vi "WPI_CANJaguar_GetStatus.vi"(8 "error in (no error)":errorcluster, 9 "Force On-Demand":bool, 10 "Status Select":T1[](array[typedef])=[enum."Output Voltage"], 11 "CAN Jaguar Ref":T3={"DeviceStatus"={"status"=FALSE, "code"=0, "source"=""}, "Type"=enum."PWM", "PWM"={"PWM Channel"=enum."PWM 1", "DeadBand"={"Name"="", "maxPositivePwm"=0, "minPositivePwm"=0, "centerPwm"=0, "maxNegativePwm"=0, "minNegativePwm"=0, "angularRange"=0}}, "CAN"={"Device Number"=0, "SetOutput VI Ref"=variant(enum8{"Percent VBus", "Current", "Speed", "Position", "Voltage"} enum."Percent VBus"), "GetOutput VI Ref"=variant(refnum<k1> refnum), "Enable VI Ref"=variant(dbl 12.0), "Disable VI Ref"=variant(enum8{"Percent VBus", "Speed", "Position", "Slave", "Unchanged / Invalid", "Voltage Compensation", "Current", "Motion Profile"} enum."Percent VBus"), "Data"=variant}, "Invert"=FALSE}) -> (0 "error out":errorcluster, 2 "Status":T2 {"Fault Counters"."CAN Status" format="%.0x"}, 3 "CAN Jaguar Ref":T3={"DeviceStatus"={"status"=FALSE, "code"=0, "source"=""}, "Type"=enum."PWM", "PWM"={"PWM Channel"=enum."PWM 1", "DeadBand"={"Name"="", "maxPositivePwm"=0, "minPositivePwm"=0, "centerPwm"=0, "maxNegativePwm"=0, "minNegativePwm"=0, "angularRange"=0}}, "CAN"={"Device Number"=0, "SetOutput VI Ref"=variant(enum8{"Percent VBus", "Current", "Speed", "Position", "Voltage"} enum."Percent VBus"), "GetOutput VI Ref"=variant(refnum<k1> refnum), "Enable VI Ref"=variant(dbl 12.0), "Disable VI Ref"=variant(enum8{"Percent VBus", "Speed", "Position", "Slave", "Unchanged / Invalid", "Voltage Compensation", "Current", "Motion Profile"} enum."Percent VBus"), "Data"=variant}, "Invert"=FALSE})   [LabVIEW 2016]
doc: "Read status information from a CAN Jaguar.\n\nThis VI allows you to specify which parts of the status you care about so that you do not waste CAN bus bandwidth. Use this VI to read status <B>On Demand</B> or status that is already received on a <B>Periodic Status Channel</B>.\n\nAll outputs are in engineering units (Volts, Amps, degrees Celsius, Rotations, and Rotations per Minute)\n\nSticky outputs are faults or limits that have occurred since the last time they were read, but may not be the current condition."
uses:
  <vilib>/Rock Robotics/WPI/MotorControl/WPI_MotorControlDeviceRef.ctl
  <vilib>/Rock Robotics/WPI/MotorControl/WPI_MotorControlType.ctl
  <vilib>/Rock Robotics/SystemInterfaces/DIO/FPGA_DIOPWMChannel.ctl
  <vilib>/Rock Robotics/WPI/PWM/WPI_PWMDeadband.ctl
  <vilib>/Rock Robotics/WPI/ThirdParty/CanMotor/CAN Jaguar/SubVIs/WPI_CANJaguar_Status.ctl
  <vilib>/Rock Robotics/WPI/ThirdParty/CanMotor/CAN Jaguar/SubVIs/WPI_CANJaguar_StatusSelect.ctl
  <vilib>/Rock Robotics/WPI/ThirdParty/CanMotor/CAN Jaguar/SubVIs/WPI_CANJaguar_StatusChannelSelect.ctl
  <vilib>/Rock Robotics/WPI/ThirdParty/CanMotor/CAN Jaguar/SubVIs/WPI_CAN_SystemMessageIDs.ctl
  <vilib>/Rock Robotics/WPI/ThirdParty/CanMotor/CAN Jaguar/SubVIs/WPI_CAN_MotorMessageIDs.ctl
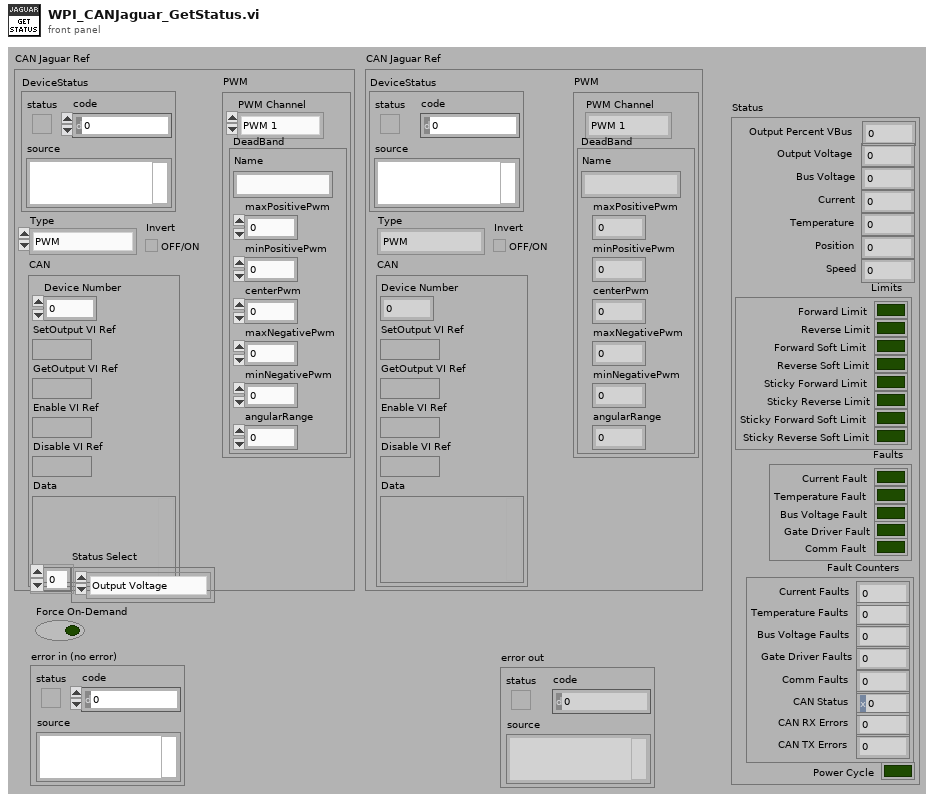
[diagram p1: front panel]
types:
  T1 = typedef "WPI_CANJaguar_StatusSelect.ctl" = enum16{"Output Percent VBus", "Output Voltage", "Bus Voltage", "Current", "Temperature", "Position", "Speed", "Limit Switches", "Faults", "Fault Counters", "Power Cycle"}
  T2 = typedef "WPI_CANJaguar_Status.ctl" = cluster{"Output Percent VBus":dbl, "Output Voltage":dbl, "Bus Voltage":dbl, "Current":dbl, "Temperature":dbl, "Position":dbl, "Speed":dbl, "Limits":cluster{"Forward Limit":bool, "Reverse Limit":bool, "Forward Soft Limit":bool, "Reverse Soft Limit":bool, "Sticky Forward Limit":bool, "Sticky Reverse Limit":bool, "Sticky Forward Soft Limit":bool, "Sticky Reverse Soft Limit":bool}, "Faults":cluster{"Current Fault":bool, "Temperature Fault":bool, "Bus Voltage Fault":bool, "Gate Driver Fault":bool, "Comm Fault":bool}, "Fault Counters":cluster{"Current Faults":u8, "Temperature Faults":u8, "Bus Voltage Faults":u8, "Gate Driver Faults":u8, "Comm Faults":u8, "CAN Status":u8, "CAN RX Errors":u8, "CAN TX Errors":u8}, "Power Cycle":bool}
  T3 = typedef "WPI_MotorControlDeviceRef.ctl" = cluster{"DeviceStatus":errorcluster, "Type":T4, "PWM":cluster{"PWM Channel":T5, "DeadBand":T6}, "CAN":cluster{"Device Number":u8, "SetOutput VI Ref":variant, "GetOutput VI Ref":variant, "Enable VI Ref":variant, "Disable VI Ref":variant, "Data":variant}, "Invert":bool}
  T4 = typedef "WPI_MotorControlType.ctl" = enum16{"PWM", "CAN"}
  T5 = typedef "FPGA_DIOPWMChannel.ctl" = enum8{"PWM 0", "PWM 1", "PWM 2", "PWM 3", "PWM 4", "PWM 5", "PWM 6", "PWM 7", "PWM 8", "PWM 9", "PWM MXP 0", "PWM MXP 1", "PWM MXP 2", "PWM MXP 3", "PWM MXP 4", "PWM MXP 5", "PWM MXP 6", "PWM MXP 7", "PWM MXP 8", "PWM MXP 9", "Invalid"}
  T6 = typedef "WPI_PWMDeadband.ctl" = cluster{"Name":string, "maxPositivePwm":i32, "minPositivePwm":i32, "centerPwm":i32, "maxNegativePwm":i32, "minNegativePwm":i32, "angularRange":u16}
  T7 = typedef "WPI_CANJaguar_StatusChannelSelect.ctl" = enum16{"Periodic Status Channel 1", "Periodic Status Channel 2", "Periodic Status Channel 3", "Periodic Status Channel 4", "On Demand Status"}
  T8 = enum16{"big-endian, network order", "native, host order", "little-endian"}
  T9 = typedef "WPI_CAN_PeriodicStatusIDs.ctl" = enum16{"Disabled", "Percent VBus Out (Byte 0)", "Percent VBus Out (Byte 1)", "VBus (Byte 0)", "VBus (Byte 1)", "Current (Byte 0)", "Current (Byte 1)", "Temperature (Byte 0)", "Temperature (Byte 1)", "Position (Byte 0)", "Position (Byte 1)", "Position (Byte 2)", "Position (Byte 3)", "Speed (Byte 0)", "Speed (Byte 1)", "Speed (Byte 2)", "Speed (Byte 3)", "Limit Switches (No Clear)", "Limit Switches (Clear)", "Faults", "Sticky Faults (No Clear)", "Sticky Faults (Clear)", "Volts Out (Byte 0)", "Volts Out (Byte 1)", "Current Fault Counter", "Temperature Fault Counter", "VBus Fault Counter", "Gate Driver Fault Counter", "Comm Fault Counter", "CANSTS", "CANERR (Byte 0)", "CANERR (Byte 1)", "Power Cycle"}
  T10 = typedef "WPI_CAN_SystemMessageIDs.ctl" = u32
  T11 = typedef "WPI_CAN_MotorMessageIDs.ctl" = u32
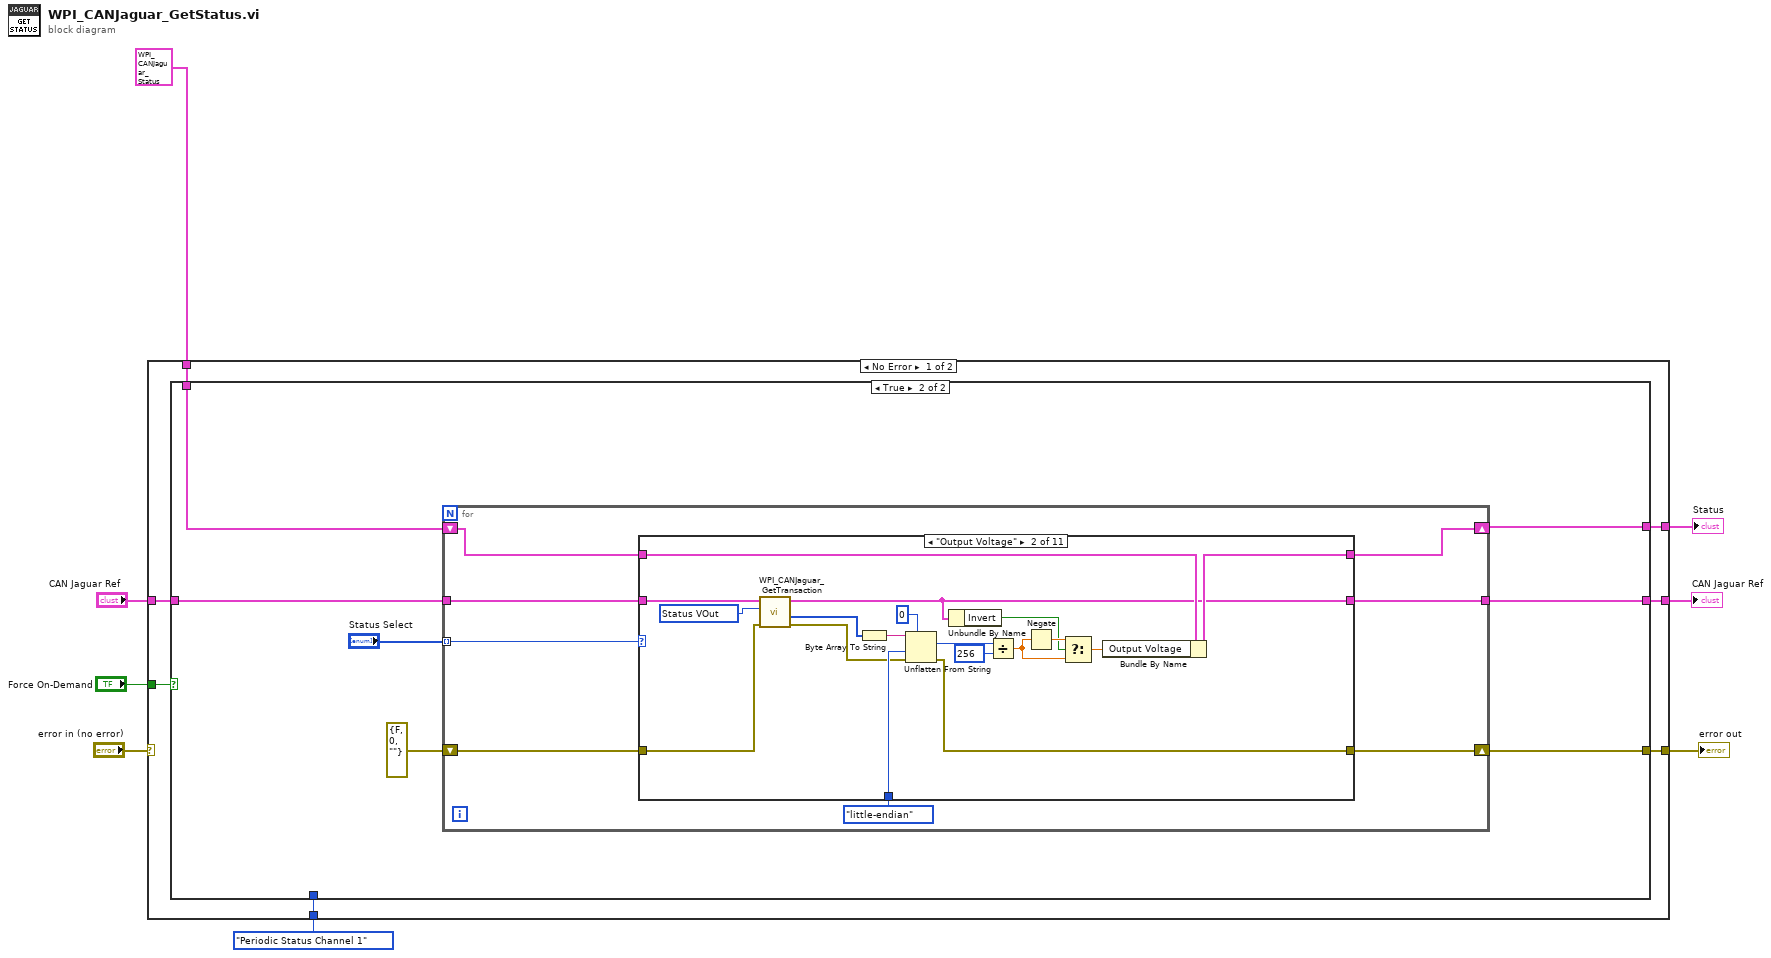
[diagram p0: block diagram]
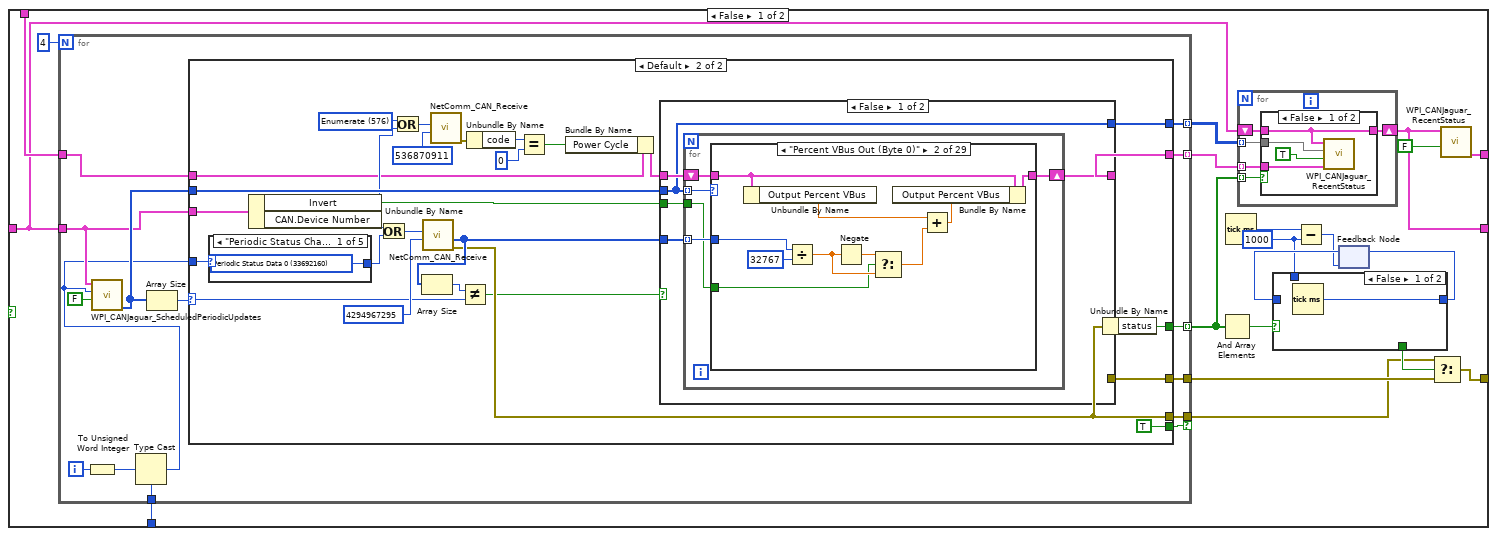
[diagram p2: hidden frame]
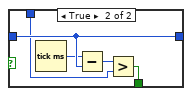
[diagram p3: hidden frame]
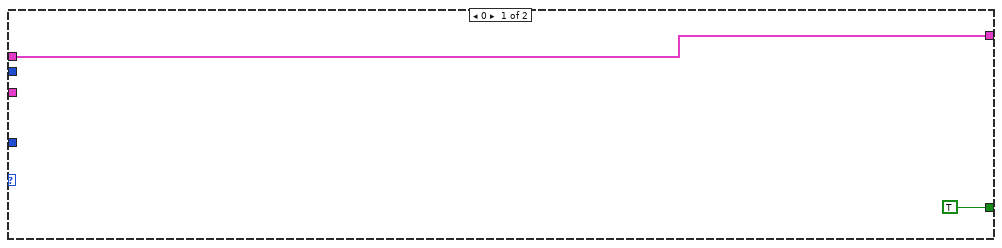
[diagram p5: hidden frame]
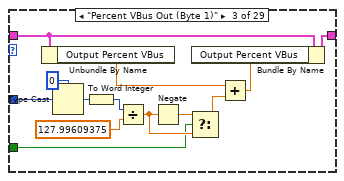
[diagram p7: hidden frame]
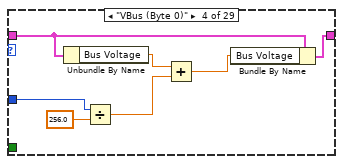
[diagram p8: hidden frame]
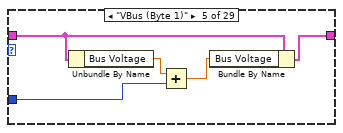
[diagram p9: hidden frame]
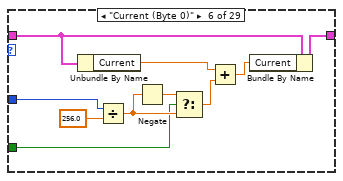
[diagram p10: hidden frame]
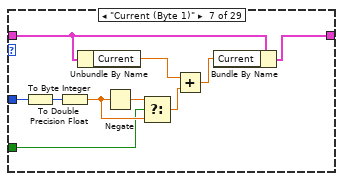
[diagram p11: hidden frame]
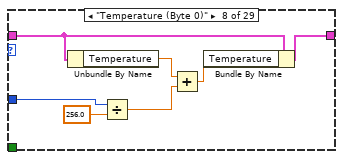
[diagram p12: hidden frame]
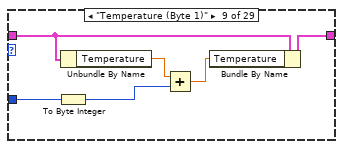
[diagram p13: hidden frame]
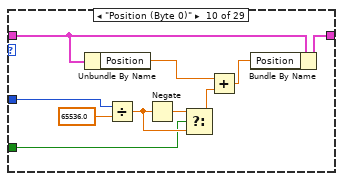
[diagram p14: hidden frame]
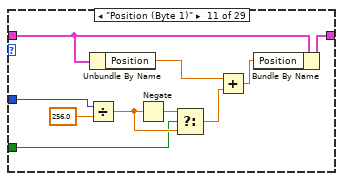
[diagram p15: hidden frame]
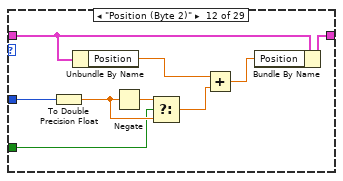
[diagram p16: hidden frame]
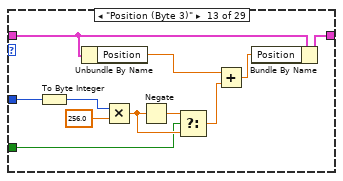
[diagram p17: hidden frame]
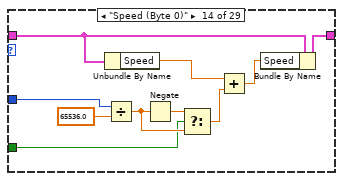
[diagram p18: hidden frame]
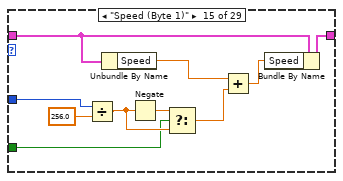
[diagram p19: hidden frame]
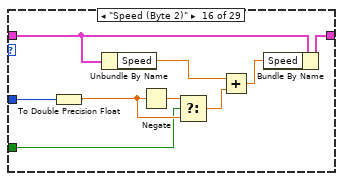
[diagram p20: hidden frame]
diagram:
  n1 = case shown="No Error" "error in (no error)" {
    selector: "error in (no error)" -> [_ w550]
    tunnel: [w13 w548] -> w8
    tunnel: "CAN Jaguar Ref" -> [w14 w548]
    tunnel: [w15 w550] -> w6
    tunnel: T2 {"Output Percent VBus"=0.0, "Output Voltage"=0.0, "Bus Voltage"=0.0, "Current"=0.0, "Temperature"=0.0, "Position"=0.0, "Speed"=0.0, "Limits"={"Forward Limit"=FALSE, "Reverse Limit"=FALSE, "Forward Soft Limit"=FALSE, "Reverse Soft Limit"=FALSE, "Sticky Forward Limit"=FALSE, "Sticky Reverse Limit"=FALSE, "Sticky Forward Soft Limit"=FALSE, "Sticky Reverse Soft Limit"=FALSE}, "Faults"={"Current Fault"=FALSE, "Temperature Fault"=FALSE, "Bus Voltage Fault"=FALSE, "Gate Driver Fault"=FALSE, "Comm Fault"=FALSE}, "Fault Counters"={"Current Faults"=0, "Temperature Faults"=0, "Bus Voltage Faults"=0, "Gate Driver Faults"=0, "Comm Faults"=0, "CAN Status"=0, "CAN RX Errors"=0, "CAN TX Errors"=0}, "Power Cycle"=FALSE} ("Status") -> [w12 w549]
    tunnel: [w11 w549] -> w3
    tunnel: "Force On-Demand" -> [w10 _]
    tunnel: WPI_CANJaguar_StatusChannelSelect."Periodic Status Channel 1" ("Status Channel Select") -> [w9 _]
    frame No Error {
      n2 = case shown="True" w10 {
        tunnel: [w17 w334] -> w15
        tunnel: w14 -> [w28 w332]
        tunnel: [w27 w331] -> w13
        tunnel: w12 -> [w35 w330]
        tunnel: [w31 w329] -> w11
        tunnel: w9 -> [w33 _]
        frame False {
          w20 = u32 1000 ("y")
          n3 = for {
            N: 4 -> [_]
            tunnel: [w63] -> w18
            tunnel: w28 -> [w60]
            tunnel: w33 -> [w56]
            tunnel: [w55] -> w26 mode=indexing
            tunnel: w35 -> [w66]
            tunnel: [w65] -> w30 mode=indexing
            tunnel: [w54] -> w29 mode=indexing
            tunnel: [w53] -> w16 if=w52
            i -> [w59]
            n4 = To Unsigned Word Integer(number=w59) -> (unsigned 16bit integer=w57:u16)
            n5 = Type Cast(type=w56, x=w57) -> (*(type *) &x=w58:T7)
            n6 = call <vilib>:"WPI_CANJaguar_ScheduledPeriodicUpdates.vi"("Update"=FALSE, "Status Channel Select"=w58, "CAN Jaguar Ref"=w60) -> ("Fields Out"=w62:T9[])  [unwired: 8 in]
            n7 = Array Size(array=w62) -> (size(s)=w64:i32)
            n8 = case shown="Default" w64 {
              selector: w64 -> [_ w91]
              tunnel: w58 -> [_ w71]
              tunnel: w62 -> [_ w89]
              tunnel: w66 -> [w68 w79]
              tunnel: [w68 w76] -> w65
              tunnel: w60 -> [_ w87]
              tunnel: [_ w90] -> w63
              tunnel: [TRUE ("status") w74] -> w55
              tunnel: [_ w75] -> w54
              tunnel: [_ w73] -> w53
              tunnel: [_ TRUE ("status")] -> w52
              frame 0 {
              }
              frame Default {
                w85 = T10 576 items=["Device Assignment"=128, "Device Query"=192, "Sync Update"=384, "Firmware Update"=448, "Firmware Version"=512, "Enumerate"=576] ("CAN System Message IDs")
                n9 = case shown="\"Periodic Status Channel 1\"" w71 {
                  tunnel: [w324 w325 w326 w327 _] -> w95
                  frame "Periodic Status Channel 1" {
                    w324 = T11 33692160 items=["Volt Enable"=33685504, "Volt Disable"=33685568, "Volt Set"=33685632, "Volt Set Ramp"=33685696, "Volt Set No Ack"=33686080, "Speed Enable"=33686528, "Speed Disable"=33686592, "Speed Set"=33686656, "Speed P"=33686720, "Speed I"=33686784, "Speed D"=33686848, "Speed Ref"=33686912, "Speed Set No Ack"=33687232, "Volt Comp Enable"=33687552, "Volt Comp Disable"=33687616, "Volt Comp Set"=33687680, "Volt Comp In Ramp"=33687744, "Volt Comp Comp Ramp"=33687808, "Volt Comp Set No Ack"=33688128, "Position Enable"=33688576, "Position Disable"=33688640, "Position Set"=33688704, "Position P"=33688768, "Position I"=33688832, "Position D"=33688896, "Position Ref"=33688960, "Position Set No Ack"=33689280, "Current Enable"=33689600, "Current Disable"=33689664, "Current Set"=33689728, "Current P"=33689792, "Current I"=33689856, "Current D"=33689920, "Current Set No Ack"=33690240, "Status Percent VBus"=33690624, "Status VBus"=33690688, "Status Current"=33690752, "Status Temp"=33690816, "Status Position"=33690880, "Status Speed"=33690944, "Status Limit"=33691008, "Status Fault"=33691072, "Status Power"=33691136, "Status Control Mode"=33691200, "Status VOut"=33691264, "Status Sticky Fault"=33691328, "Status Fault Count"=33691392, "Periodic Status Enable 0"=33691648, "Periodic Status Enable 1"=33691712, "Periodic Status Enable 2"=33691776, "Periodic Status Enable 3"=33691840, "Periodic Status Config 0"=33691904, "Periodic Status Config 1"=33691968, "Periodic Status Config 2"=33692032, "Periodic Status Config 3"=33692096, "Periodic Status Data 0"=33692160, "Periodic Status Data 1"=33692224, "Periodic Status Data 2"=33692288, "Periodic Status Data 3"=33692352, "Config Num Brushes"=33692672, "Config Encoder Lines"=33692736, "Config Pot Turns"=33692800, "Config Brake Coast"=33692864, "Config Limit Mode"=33692928, "Config Limit Fwd"=33692992, "Config Limit Rev"=33693056, "Config Max VOut"=33693120, "Config Fault Time"=33693184, "Motor Ack"=33693696] ("CAN Motor Message IDs")
                  }
                  frame "Periodic Status Channel 2" {
                    w325 = T11 33692224 items=["Volt Enable"=33685504, "Volt Disable"=33685568, "Volt Set"=33685632, "Volt Set Ramp"=33685696, "Volt Set No Ack"=33686080, "Speed Enable"=33686528, "Speed Disable"=33686592, "Speed Set"=33686656, "Speed P"=33686720, "Speed I"=33686784, "Speed D"=33686848, "Speed Ref"=33686912, "Speed Set No Ack"=33687232, "Volt Comp Enable"=33687552, "Volt Comp Disable"=33687616, "Volt Comp Set"=33687680, "Volt Comp In Ramp"=33687744, "Volt Comp Comp Ramp"=33687808, "Volt Comp Set No Ack"=33688128, "Position Enable"=33688576, "Position Disable"=33688640, "Position Set"=33688704, "Position P"=33688768, "Position I"=33688832, "Position D"=33688896, "Position Ref"=33688960, "Position Set No Ack"=33689280, "Current Enable"=33689600, "Current Disable"=33689664, "Current Set"=33689728, "Current P"=33689792, "Current I"=33689856, "Current D"=33689920, "Current Set No Ack"=33690240, "Status Percent VBus"=33690624, "Status VBus"=33690688, "Status Current"=33690752, "Status Temp"=33690816, "Status Position"=33690880, "Status Speed"=33690944, "Status Limit"=33691008, "Status Fault"=33691072, "Status Power"=33691136, "Status Control Mode"=33691200, "Status VOut"=33691264, "Status Sticky Fault"=33691328, "Status Fault Count"=33691392, "Periodic Status Enable 0"=33691648, "Periodic Status Enable 1"=33691712, "Periodic Status Enable 2"=33691776, "Periodic Status Enable 3"=33691840, "Periodic Status Config 0"=33691904, "Periodic Status Config 1"=33691968, "Periodic Status Config 2"=33692032, "Periodic Status Config 3"=33692096, "Periodic Status Data 0"=33692160, "Periodic Status Data 1"=33692224, "Periodic Status Data 2"=33692288, "Periodic Status Data 3"=33692352, "Config Num Brushes"=33692672, "Config Encoder Lines"=33692736, "Config Pot Turns"=33692800, "Config Brake Coast"=33692864, "Config Limit Mode"=33692928, "Config Limit Fwd"=33692992, "Config Limit Rev"=33693056, "Config Max VOut"=33693120, "Config Fault Time"=33693184, "Motor Ack"=33693696] ("CAN Motor Message IDs")
                  }
                  frame "Periodic Status Channel 3" {
                    w326 = T11 33692288 items=["Volt Enable"=33685504, "Volt Disable"=33685568, "Volt Set"=33685632, "Volt Set Ramp"=33685696, "Volt Set No Ack"=33686080, "Speed Enable"=33686528, "Speed Disable"=33686592, "Speed Set"=33686656, "Speed P"=33686720, "Speed I"=33686784, "Speed D"=33686848, "Speed Ref"=33686912, "Speed Set No Ack"=33687232, "Volt Comp Enable"=33687552, "Volt Comp Disable"=33687616, "Volt Comp Set"=33687680, "Volt Comp In Ramp"=33687744, "Volt Comp Comp Ramp"=33687808, "Volt Comp Set No Ack"=33688128, "Position Enable"=33688576, "Position Disable"=33688640, "Position Set"=33688704, "Position P"=33688768, "Position I"=33688832, "Position D"=33688896, "Position Ref"=33688960, "Position Set No Ack"=33689280, "Current Enable"=33689600, "Current Disable"=33689664, "Current Set"=33689728, "Current P"=33689792, "Current I"=33689856, "Current D"=33689920, "Current Set No Ack"=33690240, "Status Percent VBus"=33690624, "Status VBus"=33690688, "Status Current"=33690752, "Status Temp"=33690816, "Status Position"=33690880, "Status Speed"=33690944, "Status Limit"=33691008, "Status Fault"=33691072, "Status Power"=33691136, "Status Control Mode"=33691200, "Status VOut"=33691264, "Status Sticky Fault"=33691328, "Status Fault Count"=33691392, "Periodic Status Enable 0"=33691648, "Periodic Status Enable 1"=33691712, "Periodic Status Enable 2"=33691776, "Periodic Status Enable 3"=33691840, "Periodic Status Config 0"=33691904, "Periodic Status Config 1"=33691968, "Periodic Status Config 2"=33692032, "Periodic Status Config 3"=33692096, "Periodic Status Data 0"=33692160, "Periodic Status Data 1"=33692224, "Periodic Status Data 2"=33692288, "Periodic Status Data 3"=33692352, "Config Num Brushes"=33692672, "Config Encoder Lines"=33692736, "Config Pot Turns"=33692800, "Config Brake Coast"=33692864, "Config Limit Mode"=33692928, "Config Limit Fwd"=33692992, "Config Limit Rev"=33693056, "Config Max VOut"=33693120, "Config Fault Time"=33693184, "Motor Ack"=33693696] ("CAN Motor Message IDs")
                  }
                  frame "Periodic Status Channel 4" {
                    w327 = T11 33692352 items=["Volt Enable"=33685504, "Volt Disable"=33685568, "Volt Set"=33685632, "Volt Set Ramp"=33685696, "Volt Set No Ack"=33686080, "Speed Enable"=33686528, "Speed Disable"=33686592, "Speed Set"=33686656, "Speed P"=33686720, "Speed I"=33686784, "Speed D"=33686848, "Speed Ref"=33686912, "Speed Set No Ack"=33687232, "Volt Comp Enable"=33687552, "Volt Comp Disable"=33687616, "Volt Comp Set"=33687680, "Volt Comp In Ramp"=33687744, "Volt Comp Comp Ramp"=33687808, "Volt Comp Set No Ack"=33688128, "Position Enable"=33688576, "Position Disable"=33688640, "Position Set"=33688704, "Position P"=33688768, "Position I"=33688832, "Position D"=33688896, "Position Ref"=33688960, "Position Set No Ack"=33689280, "Current Enable"=33689600, "Current Disable"=33689664, "Current Set"=33689728, "Current P"=33689792, "Current I"=33689856, "Current D"=33689920, "Current Set No Ack"=33690240, "Status Percent VBus"=33690624, "Status VBus"=33690688, "Status Current"=33690752, "Status Temp"=33690816, "Status Position"=33690880, "Status Speed"=33690944, "Status Limit"=33691008, "Status Fault"=33691072, "Status Power"=33691136, "Status Control Mode"=33691200, "Status VOut"=33691264, "Status Sticky Fault"=33691328, "Status Fault Count"=33691392, "Periodic Status Enable 0"=33691648, "Periodic Status Enable 1"=33691712, "Periodic Status Enable 2"=33691776, "Periodic Status Enable 3"=33691840, "Periodic Status Config 0"=33691904, "Periodic Status Config 1"=33691968, "Periodic Status Config 2"=33692032, "Periodic Status Config 3"=33692096, "Periodic Status Data 0"=33692160, "Periodic Status Data 1"=33692224, "Periodic Status Data 2"=33692288, "Periodic Status Data 3"=33692352, "Config Num Brushes"=33692672, "Config Encoder Lines"=33692736, "Config Pot Turns"=33692800, "Config Brake Coast"=33692864, "Config Limit Mode"=33692928, "Config Limit Fwd"=33692992, "Config Limit Rev"=33693056, "Config Max VOut"=33693120, "Config Fault Time"=33693184, "Motor Ack"=33693696] ("CAN Motor Message IDs")
                  }
                  frame Default {
                  }
                }
                n10 = Unbundle By Name(w87) -> ("Invert"=w88:bool, "CAN.Device Number"=w80:u8)
                n11 = Or(x=w80, y=w95) -> (x .or. y?=w94:T11)
                n12 = Or(x=w85, y=w80) -> (x .or. y?=w84:T10)
                n13 = call <vilib>:"NetComm_CAN_Receive.vi"("Message ID Mask"=u32 4294967295 ("Timeout (ms)"), "Message ID"=w94) -> ("error out"=w73:errorcluster, "Data"=w92:u8[])  [unwired: 1 in, 7 out]
                n14 = Array Size(array=w92) -> (size(s)=w69:i32)
                n15 = call <vilib>:"NetComm_CAN_Receive.vi"("Message ID Mask"=u32 536870911, "Message ID"=w84) -> ("error out"=w83:errorcluster)  [unwired: 1 in, 8 out]
                n16 = Not Equal?(x=w69, y=w91) -> (x != y?=w70:bool)
                n17 = Unbundle By Name(w83) -> ("code"=w82:i32)
                n18 = Equal?(x=w82, y=0) -> (x = y?=w77:bool)
                n19 = Bundle By Name(cluster=w79, "Power Cycle"=w77) -> (w78:T2)
                n20 = case shown="False" w70 {
                  tunnel: w92 -> [w100 _]
                  tunnel: w78 -> [w99 w320]
                  tunnel: [w98 w320] -> w76
                  tunnel: w89 -> [w97 _]
                  tunnel: [_ w321] -> w90
                  tunnel: [w97 _] -> w75
                  tunnel: w88 -> [w96 _]
                  frame False {
                    n21 = for {
                      tunnel: w100 -> [w102] mode=indexing
                      tunnel: w97 -> [w105] mode=indexing
                      shift-right: [w104] -> w98
                      shift-left: w99 -> [w103]
                      tunnel: w96 -> [w101]
                      n22 = case shown="\"Percent VBus Out (Byte 0)\"" w105 {
                        tunnel: [w106 w116 w129 w136 w140 w150 w157 w163 w170 w180 w189 w199 w209 w220 w230 w240 w250 w263 w274 w281 w292 w297 w300 w303 w306 w309 w312 w315 w318] -> w104
                        tunnel: w103 -> [w106 w115 w128 w135 w141 w151 w158 w162 w171 w181 w190 w200 w210 w221 w231 w241 w251 w264 w275 w282 w293 w298 w301 w304 w307 w310 w313 w316 w319]
                        tunnel: w102 -> [_ w112 w125 w131 w138 w146 w159 w164 w172 w179 w191 w201 w211 w219 w229 w239 w249 w266 w272 w280 w291 w296 w299 w302 w305 w308 w311 w314 w317]
                        tunnel: w101 -> [_ w108 w117 _ _ w142 w153 _ _ w175 w185 w195 w205 w215 w225 w235 w245 _ _ w276 w287 _ _ _ _ _ _ _ _]
                        frame "Disabled", Default {
                        }
                        frame "Percent VBus Out (Byte 0)" {
                          n23 = Unbundle By Name(w115) -> ("Output Percent VBus"=w114:dbl)
                          n24 = Divide(x=w112, y=i16 32767) -> (x/y=w109:dbl)
                          n25 = Negate(x=w109) -> (-x=w110:dbl)
                          n26 = Select(t=w110, s=w108, f=w109) -> (s? t:f=w107:dbl)
                          n27 = Add(x=w114, y=w107) -> (x+y=w113:dbl)
                          n28 = Bundle By Name(cluster=w115, "Output Percent VBus"=w113) -> (w116:T2)
                        }
                        frame "Percent VBus Out (Byte 1)" {
                          n29 = Unbundle By Name(w128) -> ("Output Percent VBus"=w127:dbl)
                          n30 = Type Cast(type=i8 0, x=w125) -> (*(type *) &x=w124:i8)
                          n31 = To Word Integer(number=w124) -> (16bit integer=w121:i16)
                          n32 = Divide(x=w121, y=127.99609375) -> (x/y=w119:dbl)
                          n33 = Negate(x=w119) -> (-x=w120:dbl)
                          n34 = Select(t=w120, s=w117, f=w119) -> (s? t:f=w118:dbl)
                          n35 = Add(x=w127, y=w118) -> (x+y=w126:dbl)
                          n36 = Bundle By Name(cluster=w128, "Output Percent VBus"=w126) -> (w129:T2)
                        }
                        frame "VBus (Byte 0)" {
                          n37 = Unbundle By Name(w135) -> ("Bus Voltage"=w134:dbl)
                          n38 = Divide(x=w131, y=256.0) -> (x/y=w130:dbl)
                          n39 = Add(x=w134, y=w130) -> (x+y=w133:dbl)
                          n40 = Bundle By Name(cluster=w135, "Bus Voltage"=w133) -> (w136:T2)
                        }
                        frame "VBus (Byte 1)" {
                          n41 = Unbundle By Name(w141) -> ("Bus Voltage"=w139:dbl)
                          n42 = Add(x=w139, y=w138) -> (x+y=w137:dbl)
                          n43 = Bundle By Name(cluster=w141, "Bus Voltage"=w137) -> (w140:T2)
                        }
                        frame "Current (Byte 0)" {
                          n44 = Unbundle By Name(w151) -> ("Current"=w149:dbl)
                          n45 = Divide(x=w146, y=256.0) -> (x/y=w144:dbl)
                          n46 = Negate(x=w144) -> (-x=w145:dbl)
                          n47 = Select(t=w145, s=w142, f=w144) -> (s? t:f=w143:dbl)
                          n48 = Add(x=w149, y=w143) -> (x+y=w148:dbl)
                          n49 = Bundle By Name(cluster=w151, "Current"=w148) -> (w150:T2)
                        }
                        frame "Current (Byte 1)" {
                          n50 = To Byte Integer(number=w159) -> (8bit integer=w152:i8)
                          n51 = To Double Precision Float(number=w152) -> (double precision float=w154:dbl)
                          n52 = Unbundle By Name(w158) -> ("Current"=w161:dbl)
                          n53 = Negate(x=w154) -> (-x=w156:dbl)
                          n54 = Select(t=w156, s=w153, f=w154) -> (s? t:f=w155:dbl)
                          n55 = Add(x=w161, y=w155) -> (x+y=w160:dbl)
                          n56 = Bundle By Name(cluster=w158, "Current"=w160) -> (w157:T2)
                        }
                        frame "Temperature (Byte 0)" {
                          n57 = Unbundle By Name(w162) -> ("Temperature"=w168:dbl)
                          n58 = Divide(x=w164, y=256.0) -> (x/y=w165:dbl)
                          n59 = Add(x=w168, y=w165) -> (x+y=w167:dbl)
                          n60 = Bundle By Name(cluster=w162, "Temperature"=w167) -> (w163:T2)
                        }
                        frame "Temperature (Byte 1)" {
                          n61 = To Byte Integer(number=w172) -> (8bit integer=w169:i8)
                          n62 = Unbundle By Name(w171) -> ("Temperature"=w174:dbl)
                          n63 = Add(x=w174, y=w169) -> (x+y=w173:dbl)
                          n64 = Bundle By Name(cluster=w171, "Temperature"=w173) -> (w170:T2)
                        }
                        frame "Position (Byte 0)" {
                          n65 = Unbundle By Name(w181) -> ("Position"=w184:dbl)
                          n66 = Divide(x=w179, y=65536.0) -> (x/y=w177:dbl)
                          n67 = Negate(x=w177) -> (-x=w178:dbl)
                          n68 = Select(t=w178, s=w175, f=w177) -> (s? t:f=w176:dbl)
                          n69 = Add(x=w184, y=w176) -> (x+y=w183:dbl)
                          n70 = Bundle By Name(cluster=w181, "Position"=w183) -> (w180:T2)
                        }
                        frame "Position (Byte 1)" {
                          n71 = Divide(x=w191, y=256.0) -> (x/y=w187:dbl)
                          n72 = Unbundle By Name(w190) -> ("Position"=w194:dbl)
                          n73 = Negate(x=w187) -> (-x=w188:dbl)
                          n74 = Select(t=w188, s=w185, f=w187) -> (s? t:f=w186:dbl)
                          n75 = Add(x=w194, y=w186) -> (x+y=w193:dbl)
                          n76 = Bundle By Name(cluster=w190, "Position"=w193) -> (w189:T2)
                        }
                        frame "Position (Byte 2)" {
                          n77 = To Double Precision Float(number=w201) -> (double precision float=w197:dbl)
                          n78 = Unbundle By Name(w200) -> ("Position"=w203:dbl)
                          n79 = Negate(x=w197) -> (-x=w198:dbl)
                          n80 = Select(t=w198, s=w195, f=w197) -> (s? t:f=w196:dbl)
                          n81 = Add(x=w203, y=w196) -> (x+y=w202:dbl)
                          n82 = Bundle By Name(cluster=w200, "Position"=w202) -> (w199:T2)
                        }
                        frame "Position (Byte 3)" {
                          n83 = To Byte Integer(number=w211) -> (8bit integer=w204:i8)
                          n84 = Unbundle By Name(w210) -> ("Position"=w214:dbl)
                          n85 = Multiply(x=w204, y=256.0) -> (x*y=w207:dbl)
                          n86 = Negate(x=w207) -> (-x=w208:dbl)
                          n87 = Select(t=w208, s=w205, f=w207) -> (s? t:f=w206:dbl)
                          n88 = Add(x=w214, y=w206) -> (x+y=w213:dbl)
                          n89 = Bundle By Name(cluster=w210, "Position"=w213) -> (w209:T2)
                        }
                        frame "Speed (Byte 0)" {
                          n90 = Unbundle By Name(w221) -> ("Speed"=w224:dbl)
                          n91 = Divide(x=w219, y=65536.0) -> (x/y=w217:dbl)
                          n92 = Negate(x=w217) -> (-x=w218:dbl)
                          n93 = Select(t=w218, s=w215, f=w217) -> (s? t:f=w216:dbl)
                          n94 = Add(x=w224, y=w216) -> (x+y=w223:dbl)
                          n95 = Bundle By Name(cluster=w221, "Speed"=w223) -> (w220:T2)
                        }
                        frame "Speed (Byte 1)" {
                          n96 = Divide(x=w229, y=256.0) -> (x/y=w227:dbl)
                          n97 = Unbundle By Name(w231) -> ("Speed"=w234:dbl)
                          n98 = Negate(x=w227) -> (-x=w228:dbl)
                          n99 = Select(t=w228, s=w225, f=w227) -> (s? t:f=w226:dbl)
                          n100 = Add(x=w234, y=w226) -> (x+y=w233:dbl)
                          n101 = Bundle By Name(cluster=w231, "Speed"=w233) -> (w230:T2)
                        }
                        frame "Speed (Byte 2)" {
                          n102 = To Double Precision Float(number=w239) -> (double precision float=w237:dbl)
                          n103 = Unbundle By Name(w241) -> ("Speed"=w243:dbl)
                          n104 = Negate(x=w237) -> (-x=w238:dbl)
                          n105 = Select(t=w238, s=w235, f=w237) -> (s? t:f=w236:dbl)
                          n106 = Add(x=w243, y=w236) -> (x+y=w242:dbl)
                          n107 = Bundle By Name(cluster=w241, "Speed"=w242) -> (w240:T2)
                        }
                        frame "Speed (Byte 3)" {
                          n108 = To Byte Integer(number=w249) -> (8bit integer=w244:i8)
                          n109 = Multiply(x=w244, y=256.0) -> (x*y=w247:dbl)
                          n110 = Unbundle By Name(w251) -> ("Speed"=w254:dbl)
                          n111 = Negate(x=w247) -> (-x=w248:dbl)
                          n112 = Select(t=w248, s=w245, f=w247) -> (s? t:f=w246:dbl)
                          n113 = Add(x=w254, y=w246) -> (x+y=w253:dbl)
                          n114 = Bundle By Name(cluster=w251, "Speed"=w253) -> (w250:T2)
                        }
                        frame "Limit Switches (No Clear)", "Limit Switches (Clear)" {
                          n115 = Number To Boolean Array(number=w266) -> (Boolean array=w265:bool[])
                          n116 = Index Array(array=w265) -> (element #1=w262:bool, element #2=w261:bool, element #3=w260:bool, element #4=w259:bool, element #5=w258:bool, element #6=w257:bool, element #7=w256:bool, element #8=w255:bool)  [unwired: 8 in]
                          n117 = Bundle By Name(cluster=w264, "Limits.Forward Limit"=w262, "Limits.Reverse Limit"=w261, "Limits.Forward Soft Limit"=w260, "Limits.Reverse Soft Limit"=w259, "Limits.Sticky Forward Limit"=w258, "Limits.Sticky Reverse Limit"=w257, "Limits.Sticky Forward Soft Limit"=w256, "Limits.Sticky Reverse Soft Limit"=w255) -> (w263:T2)
                        }
                        frame "Faults".."Sticky Faults (Clear)" {
                          n118 = Number To Boolean Array(number=w272) -> (Boolean array=w273:bool[])
                          n119 = Index Array(array=w273) -> (element #1=w271:bool, element #2=w270:bool, element #3=w269:bool, element #4=w268:bool, element #5=w267:bool)  [unwired: 5 in]
                          n120 = Bundle By Name(cluster=w275, "Faults.Current Fault"=w271, "Faults.Temperature Fault"=w270, "Faults.Bus Voltage Fault"=w269, "Faults.Gate Driver Fault"=w268, "Faults.Comm Fault"=w267) -> (w274:T2)
                        }
                        frame "Volts Out (Byte 0)" {
                          n121 = Unbundle By Name(w282) -> ("Output Voltage"=w285:dbl)
                          n122 = Divide(x=w280, y=256.0) -> (x/y=w278:dbl)
                          n123 = Negate(x=w278) -> (-x=w279:dbl)
                          n124 = Select(t=w279, s=w276, f=w278) -> (s? t:f=w277:dbl)
                          n125 = Add(x=w285, y=w277) -> (x+y=w284:dbl)
                          n126 = Bundle By Name(cluster=w282, "Output Voltage"=w284) -> (w281:T2)
                        }
                        frame "Volts Out (Byte 1)" {
                          n127 = To Byte Integer(number=w291) -> (8bit integer=w286:i8)
                          n128 = To Double Precision Float(number=w286) -> (double precision float=w289:dbl)
                          n129 = Unbundle By Name(w293) -> ("Output Voltage"=w295:dbl)
                          n130 = Negate(x=w289) -> (-x=w290:dbl)
                          n131 = Select(t=w290, s=w287, f=w289) -> (s? t:f=w288:dbl)
                          n132 = Add(x=w295, y=w288) -> (x+y=w294:dbl)
                          n133 = Bundle By Name(cluster=w293, "Output Voltage"=w294) -> (w292:T2)
                        }
                        frame "Current Fault Counter" {
                          n134 = Bundle By Name(cluster=w298, "Fault Counters.Current Faults"=w296) -> (w297:T2)
                        }
                        frame "Temperature Fault Counter" {
                          n135 = Bundle By Name(cluster=w301, "Fault Counters.Temperature Faults"=w299) -> (w300:T2)
                        }
                        frame "VBus Fault Counter" {
                          n136 = Bundle By Name(cluster=w304, "Fault Counters.Bus Voltage Faults"=w302) -> (w303:T2)
                        }
                        frame "Gate Driver Fault Counter" {
                          n137 = Bundle By Name(cluster=w307, "Fault Counters.Gate Driver Faults"=w305) -> (w306:T2)
                        }
                        frame "Comm Fault Counter" {
                          n138 = Bundle By Name(cluster=w310, "Fault Counters.Comm Faults"=w308) -> (w309:T2)
                        }
                        frame "CANSTS" {
                          n139 = Bundle By Name(cluster=w313, "Fault Counters.CAN Status"=w311) -> (w312:T2)
                        }
                        frame "CANERR (Byte 0)" {
                          n140 = Bundle By Name(cluster=w316, "Fault Counters.CAN RX Errors"=w314) -> (w315:T2)
                        }
                        frame "CANERR (Byte 1)" {
                          n141 = Bundle By Name(cluster=w319, "Fault Counters.CAN TX Errors"=w317) -> (w318:T2)
                        }
                      }
                    }
                  }
                  frame True {
                    # "#TODO - Not the best error code in the world..."
                    n142 = call <vilib>:"WPI_UtilitiesFRC Build Error.vi"("error code"=-44086, "extra error text"="Did not receive the appropriate number of bytes from the Jaguar.") -> ("error out"=w321:errorcluster)  [unwired: 3 in, 10 out]
                  }
                }
                n143 = Unbundle By Name(w73) -> ("status"=w74:bool)
              }
            }
          }
          n144 = And Array Elements(Boolean array=w26) -> (logical AND=w25:bool)
          n145 = Tick Count (ms)() -> (millisecond timer value=w22:u32)
          n146 = for {
            tunnel: w26 -> [w45] mode=indexing
            tunnel: w30 -> [w44] mode=indexing
            tunnel: w29 -> [w43] mode=indexing
            shift-right: [w42] -> w27
            shift-left: w28 -> [w46]
            n147 = case shown="False" w45 {
              tunnel: w44 -> [w50 _]
              tunnel: w43 -> [w48 _]
              tunnel: w46 -> [w47 w51]
              tunnel: [w47 w51] -> w42
              frame False {
                n148 = call <vilib>:"WPI_CANJaguar_RecentStatus.vi"("Status In"=w50, "Update"=TRUE, "Fields"=w48, "CAN Jaguar Ref"=w47) -> ()  [unwired: 7 in, 1 out]
              }
              frame True {
              }
            }
          }
          n149 = Subtract(x=w22, y=w20) -> (x-y=w21:u32)
          n150 = feedback #1(w21) -> (w23:u32)
          n151 = case shown="False" w25 {
            tunnel: [w36 w41] -> w24
            tunnel: w23 -> [_ w41]
            tunnel: w20 -> [_ w38]
            tunnel: [_ w37] -> w19
            frame False {
              n152 = Tick Count (ms)() -> (millisecond timer value=w36:u32)
            }
            frame True {
              n153 = Tick Count (ms)() -> (millisecond timer value=w40:u32)
              n154 = Subtract(x=w40, y=w41) -> (x-y=w39:u32)
              n155 = Greater?(x=w39, y=w38) -> (0:w37:bool)
            }
          }
          n156 = feedback-in #1(w24) -> ()
          n157 = Select(t=w16, s=w19, f=w18) -> (s? t:f=w17:errorcluster)
          n158 = call <vilib>:"WPI_CANJaguar_RecentStatus.vi"("Update"=FALSE, "CAN Jaguar Ref"=w27) -> ("Status Out"=w31:T2)  [unwired: 9 in]
        }
        frame True {
          n159 = for {
            tunnel: "Status Select" -> [w342] mode=indexing
            shift-right: [w336] -> w329
            shift-left: w330 -> [w337]
            shift-right: [w339] -> w334
            shift-left: errorcluster {"status"=FALSE, "code"=0, "source"=""} ("error out") -> [w335]
            tunnel: w332 -> [w340]
            tunnel: [w338] -> w331
            n160 = case shown="\"Output Voltage\"" w342 {
              tunnel: T8."little-endian" ("byte order (0:big-endian, network order)") -> [w353 w371 w385 w411 w426 w444 w462 w484 w503 _ w530]
              tunnel: [w360 w378 w393 w409 w424 w442 w460 w482 w485 w507 w524] -> w339
              tunnel: w337 -> [w359 w377 w392 w408 w421 w441 w459 w481 w501 w522 w539]
              tunnel: [w358 w376 w391 w407 w420 w440 w458 w480 w500 w521 w538] -> w336
              tunnel: w340 -> [w350 w368 w381 w401 w418 w433 w451 w472 w492 w517 w531]
              tunnel: [w347 w365 w383 w396 w413 w427 w445 w470 w486 w504 w528] -> w338
              tunnel: w335 -> [w349 w367 w380 w399 w412 w432 w450 w469 w491 w516 w527]
              frame "Output Percent VBus" {
                w351 = T11 33690624 items=["Volt Enable"=33685504, "Volt Disable"=33685568, "Volt Set"=33685632, "Volt Set Ramp"=33685696, "Volt Set No Ack"=33686080, "Speed Enable"=33686528, "Speed Disable"=33686592, "Speed Set"=33686656, "Speed P"=33686720, "Speed I"=33686784, "Speed D"=33686848, "Speed Ref"=33686912, "Speed Set No Ack"=33687232, "Volt Comp Enable"=33687552, "Volt Comp Disable"=33687616, "Volt Comp Set"=33687680, "Volt Comp In Ramp"=33687744, "Volt Comp Comp Ramp"=33687808, "Volt Comp Set No Ack"=33688128, "Position Enable"=33688576, "Position Disable"=33688640, "Position Set"=33688704, "Position P"=33688768, "Position I"=33688832, "Position D"=33688896, "Position Ref"=33688960, "Position Set No Ack"=33689280, "Current Enable"=33689600, "Current Disable"=33689664, "Current Set"=33689728, "Current P"=33689792, "Current I"=33689856, "Current D"=33689920, "Current Set No Ack"=33690240, "Status Percent VBus"=33690624, "Status VBus"=33690688, "Status Current"=33690752, "Status Temp"=33690816, "Status Position"=33690880, "Status Speed"=33690944, "Status Limit"=33691008, "Status Fault"=33691072, "Status Power"=33691136, "Status Control Mode"=33691200, "Status VOut"=33691264, "Status Sticky Fault"=33691328, "Status Fault Count"=33691392, "Periodic Status Enable 0"=33691648, "Periodic Status Enable 1"=33691712, "Periodic Status Enable 2"=33691776, "Periodic Status Enable 3"=33691840, "Periodic Status Config 0"=33691904, "Periodic Status Config 1"=33691968, "Periodic Status Config 2"=33692032, "Periodic Status Config 3"=33692096, "Periodic Status Data 0"=33692160, "Periodic Status Data 1"=33692224, "Periodic Status Data 2"=33692288, "Periodic Status Data 3"=33692352, "Config Num Brushes"=33692672, "Config Encoder Lines"=33692736, "Config Pot Turns"=33692800, "Config Brake Coast"=33692864, "Config Limit Mode"=33692928, "Config Limit Fwd"=33692992, "Config Limit Rev"=33693056, "Config Max VOut"=33693120, "Config Fault Time"=33693184, "Motor Ack"=33693696] ("CAN Motor Message IDs")
                n161 = call <vilib>:"WPI_CANJaguar_GetTransaction.vi"("error in"=w349, "Message ID"=w351, "CAN Jaguar Ref"=w350) -> ("error out"=w348:errorcluster, "Data Out"=w354:u8[], "CAN Jaguar Ref Out"=w347:T3)  [unwired: 6 out]
                n162 = Byte Array To String(unsigned byte array=w354) -> (string=w355:string)
                n163 = Unflatten From String(type=i16 0 ("Voltage"), binary string=w355, byte order (0:big-endian, network order)=w353, error in (no error)=w348) -> (value=w357:i16, error out=w360:errorcluster)  [unwired: 2 out]
                n164 = Unbundle By Name(w347) -> ("Invert"=w343:bool)
                n165 = Divide(x=w357, y=i16 32767) -> (x/y=w344:dbl)
                n166 = Negate(x=w344) -> (-x=w345:dbl)
                n167 = Select(t=w345, s=w343, f=w344) -> (s? t:f=w346:dbl)
                n168 = Bundle By Name(cluster=w359, "Output Percent VBus"=w346) -> (w358:T2)
              }
              frame "Output Voltage" {
                w369 = T11 33691264 items=["Volt Enable"=33685504, "Volt Disable"=33685568, "Volt Set"=33685632, "Volt Set Ramp"=33685696, "Volt Set No Ack"=33686080, "Speed Enable"=33686528, "Speed Disable"=33686592, "Speed Set"=33686656, "Speed P"=33686720, "Speed I"=33686784, "Speed D"=33686848, "Speed Ref"=33686912, "Speed Set No Ack"=33687232, "Volt Comp Enable"=33687552, "Volt Comp Disable"=33687616, "Volt Comp Set"=33687680, "Volt Comp In Ramp"=33687744, "Volt Comp Comp Ramp"=33687808, "Volt Comp Set No Ack"=33688128, "Position Enable"=33688576, "Position Disable"=33688640, "Position Set"=33688704, "Position P"=33688768, "Position I"=33688832, "Position D"=33688896, "Position Ref"=33688960, "Position Set No Ack"=33689280, "Current Enable"=33689600, "Current Disable"=33689664, "Current Set"=33689728, "Current P"=33689792, "Current I"=33689856, "Current D"=33689920, "Current Set No Ack"=33690240, "Status Percent VBus"=33690624, "Status VBus"=33690688, "Status Current"=33690752, "Status Temp"=33690816, "Status Position"=33690880, "Status Speed"=33690944, "Status Limit"=33691008, "Status Fault"=33691072, "Status Power"=33691136, "Status Control Mode"=33691200, "Status VOut"=33691264, "Status Sticky Fault"=33691328, "Status Fault Count"=33691392, "Periodic Status Enable 0"=33691648, "Periodic Status Enable 1"=33691712, "Periodic Status Enable 2"=33691776, "Periodic Status Enable 3"=33691840, "Periodic Status Config 0"=33691904, "Periodic Status Config 1"=33691968, "Periodic Status Config 2"=33692032, "Periodic Status Config 3"=33692096, "Periodic Status Data 0"=33692160, "Periodic Status Data 1"=33692224, "Periodic Status Data 2"=33692288, "Periodic Status Data 3"=33692352, "Config Num Brushes"=33692672, "Config Encoder Lines"=33692736, "Config Pot Turns"=33692800, "Config Brake Coast"=33692864, "Config Limit Mode"=33692928, "Config Limit Fwd"=33692992, "Config Limit Rev"=33693056, "Config Max VOut"=33693120, "Config Fault Time"=33693184, "Motor Ack"=33693696] ("CAN Motor Message IDs")
                n169 = call <vilib>:"WPI_CANJaguar_GetTransaction.vi"("error in"=w367, "Message ID"=w369, "CAN Jaguar Ref"=w368) -> ("error out"=w366:errorcluster, "Data Out"=w372:u8[], "CAN Jaguar Ref Out"=w365:T3)  [unwired: 6 out]
                n170 = Byte Array To String(unsigned byte array=w372) -> (string=w373:string)
                n171 = Unflatten From String(type=i16 0 ("Voltage"), binary string=w373, byte order (0:big-endian, network order)=w371, error in (no error)=w366) -> (value=w375:i16, error out=w378:errorcluster)  [unwired: 2 out]
                n172 = Unbundle By Name(w365) -> ("Invert"=w361:bool)
                n173 = Divide(x=w375, y=i16 256) -> (x/y=w362:dbl)
                n174 = Negate(x=w362) -> (-x=w363:dbl)
                n175 = Select(t=w363, s=w361, f=w362) -> (s? t:f=w364:dbl)
                n176 = Bundle By Name(cluster=w377, "Output Voltage"=w364) -> (w376:T2)
              }
              frame "Bus Voltage" {
                w382 = T11 33690688 items=["Volt Enable"=33685504, "Volt Disable"=33685568, "Volt Set"=33685632, "Volt Set Ramp"=33685696, "Volt Set No Ack"=33686080, "Speed Enable"=33686528, "Speed Disable"=33686592, "Speed Set"=33686656, "Speed P"=33686720, "Speed I"=33686784, "Speed D"=33686848, "Speed Ref"=33686912, "Speed Set No Ack"=33687232, "Volt Comp Enable"=33687552, "Volt Comp Disable"=33687616, "Volt Comp Set"=33687680, "Volt Comp In Ramp"=33687744, "Volt Comp Comp Ramp"=33687808, "Volt Comp Set No Ack"=33688128, "Position Enable"=33688576, "Position Disable"=33688640, "Position Set"=33688704, "Position P"=33688768, "Position I"=33688832, "Position D"=33688896, "Position Ref"=33688960, "Position Set No Ack"=33689280, "Current Enable"=33689600, "Current Disable"=33689664, "Current Set"=33689728, "Current P"=33689792, "Current I"=33689856, "Current D"=33689920, "Current Set No Ack"=33690240, "Status Percent VBus"=33690624, "Status VBus"=33690688, "Status Current"=33690752, "Status Temp"=33690816, "Status Position"=33690880, "Status Speed"=33690944, "Status Limit"=33691008, "Status Fault"=33691072, "Status Power"=33691136, "Status Control Mode"=33691200, "Status VOut"=33691264, "Status Sticky Fault"=33691328, "Status Fault Count"=33691392, "Periodic Status Enable 0"=33691648, "Periodic Status Enable 1"=33691712, "Periodic Status Enable 2"=33691776, "Periodic Status Enable 3"=33691840, "Periodic Status Config 0"=33691904, "Periodic Status Config 1"=33691968, "Periodic Status Config 2"=33692032, "Periodic Status Config 3"=33692096, "Periodic Status Data 0"=33692160, "Periodic Status Data 1"=33692224, "Periodic Status Data 2"=33692288, "Periodic Status Data 3"=33692352, "Config Num Brushes"=33692672, "Config Encoder Lines"=33692736, "Config Pot Turns"=33692800, "Config Brake Coast"=33692864, "Config Limit Mode"=33692928, "Config Limit Fwd"=33692992, "Config Limit Rev"=33693056, "Config Max VOut"=33693120, "Config Fault Time"=33693184, "Motor Ack"=33693696] ("CAN Motor Message IDs")
                n177 = call <vilib>:"WPI_CANJaguar_GetTransaction.vi"("error in"=w380, "Message ID"=w382, "CAN Jaguar Ref"=w381) -> ("error out"=w379:errorcluster, "Data Out"=w386:u8[], "CAN Jaguar Ref Out"=w383:T3)  [unwired: 6 out]
                n178 = Byte Array To String(unsigned byte array=w386) -> (string=w387:string)
                n179 = Unflatten From String(type=i16 0 ("Voltage"), binary string=w387, byte order (0:big-endian, network order)=w385, error in (no error)=w379) -> (value=w390:i16, error out=w393:errorcluster)  [unwired: 2 out]
                n180 = Divide(x=w390, y=i16 256) -> (x/y=w388:dbl)
                n181 = Bundle By Name(cluster=w392, "Bus Voltage"=w388) -> (w391:T2)
              }
              frame "Current" {
                w400 = T11 33690752 items=["Volt Enable"=33685504, "Volt Disable"=33685568, "Volt Set"=33685632, "Volt Set Ramp"=33685696, "Volt Set No Ack"=33686080, "Speed Enable"=33686528, "Speed Disable"=33686592, "Speed Set"=33686656, "Speed P"=33686720, "Speed I"=33686784, "Speed D"=33686848, "Speed Ref"=33686912, "Speed Set No Ack"=33687232, "Volt Comp Enable"=33687552, "Volt Comp Disable"=33687616, "Volt Comp Set"=33687680, "Volt Comp In Ramp"=33687744, "Volt Comp Comp Ramp"=33687808, "Volt Comp Set No Ack"=33688128, "Position Enable"=33688576, "Position Disable"=33688640, "Position Set"=33688704, "Position P"=33688768, "Position I"=33688832, "Position D"=33688896, "Position Ref"=33688960, "Position Set No Ack"=33689280, "Current Enable"=33689600, "Current Disable"=33689664, "Current Set"=33689728, "Current P"=33689792, "Current I"=33689856, "Current D"=33689920, "Current Set No Ack"=33690240, "Status Percent VBus"=33690624, "Status VBus"=33690688, "Status Current"=33690752, "Status Temp"=33690816, "Status Position"=33690880, "Status Speed"=33690944, "Status Limit"=33691008, "Status Fault"=33691072, "Status Power"=33691136, "Status Control Mode"=33691200, "Status VOut"=33691264, "Status Sticky Fault"=33691328, "Status Fault Count"=33691392, "Periodic Status Enable 0"=33691648, "Periodic Status Enable 1"=33691712, "Periodic Status Enable 2"=33691776, "Periodic Status Enable 3"=33691840, "Periodic Status Config 0"=33691904, "Periodic Status Config 1"=33691968, "Periodic Status Config 2"=33692032, "Periodic Status Config 3"=33692096, "Periodic Status Data 0"=33692160, "Periodic Status Data 1"=33692224, "Periodic Status Data 2"=33692288, "Periodic Status Data 3"=33692352, "Config Num Brushes"=33692672, "Config Encoder Lines"=33692736, "Config Pot Turns"=33692800, "Config Brake Coast"=33692864, "Config Limit Mode"=33692928, "Config Limit Fwd"=33692992, "Config Limit Rev"=33693056, "Config Max VOut"=33693120, "Config Fault Time"=33693184, "Motor Ack"=33693696] ("CAN Motor Message IDs")
                n182 = call <vilib>:"WPI_CANJaguar_GetTransaction.vi"("error in"=w399, "Message ID"=w400, "CAN Jaguar Ref"=w401) -> ("error out"=w402:errorcluster, "Data Out"=w403:u8[], "CAN Jaguar Ref Out"=w396:T3)  [unwired: 6 out]
                n183 = Byte Array To String(unsigned byte array=w403) -> (string=w404:string)
                n184 = Unflatten From String(type=i16 0 ("Voltage"), binary string=w404, byte order (0:big-endian, network order)=w411, error in (no error)=w402) -> (value=w406:i16, error out=w409:errorcluster)  [unwired: 2 out]
                n185 = Unbundle By Name(w396) -> ("Invert"=w398:bool)
                n186 = Divide(x=w406, y=256) -> (x/y=w394:dbl)
                n187 = Negate(x=w394) -> (-x=w397:dbl)
                n188 = Select(t=w397, s=w398, f=w394) -> (s? t:f=w395:dbl)
                n189 = Bundle By Name(cluster=w408, "Current"=w395) -> (w407:T2)
              }
              frame "Temperature" {
                w415 = T11 33690816 items=["Volt Enable"=33685504, "Volt Disable"=33685568, "Volt Set"=33685632, "Volt Set Ramp"=33685696, "Volt Set No Ack"=33686080, "Speed Enable"=33686528, "Speed Disable"=33686592, "Speed Set"=33686656, "Speed P"=33686720, "Speed I"=33686784, "Speed D"=33686848, "Speed Ref"=33686912, "Speed Set No Ack"=33687232, "Volt Comp Enable"=33687552, "Volt Comp Disable"=33687616, "Volt Comp Set"=33687680, "Volt Comp In Ramp"=33687744, "Volt Comp Comp Ramp"=33687808, "Volt Comp Set No Ack"=33688128, "Position Enable"=33688576, "Position Disable"=33688640, "Position Set"=33688704, "Position P"=33688768, "Position I"=33688832, "Position D"=33688896, "Position Ref"=33688960, "Position Set No Ack"=33689280, "Current Enable"=33689600, "Current Disable"=33689664, "Current Set"=33689728, "Current P"=33689792, "Current I"=33689856, "Current D"=33689920, "Current Set No Ack"=33690240, "Status Percent VBus"=33690624, "Status VBus"=33690688, "Status Current"=33690752, "Status Temp"=33690816, "Status Position"=33690880, "Status Speed"=33690944, "Status Limit"=33691008, "Status Fault"=33691072, "Status Power"=33691136, "Status Control Mode"=33691200, "Status VOut"=33691264, "Status Sticky Fault"=33691328, "Status Fault Count"=33691392, "Periodic Status Enable 0"=33691648, "Periodic Status Enable 1"=33691712, "Periodic Status Enable 2"=33691776, "Periodic Status Enable 3"=33691840, "Periodic Status Config 0"=33691904, "Periodic Status Config 1"=33691968, "Periodic Status Config 2"=33692032, "Periodic Status Config 3"=33692096, "Periodic Status Data 0"=33692160, "Periodic Status Data 1"=33692224, "Periodic Status Data 2"=33692288, "Periodic Status Data 3"=33692352, "Config Num Brushes"=33692672, "Config Encoder Lines"=33692736, "Config Pot Turns"=33692800, "Config Brake Coast"=33692864, "Config Limit Mode"=33692928, "Config Limit Fwd"=33692992, "Config Limit Rev"=33693056, "Config Max VOut"=33693120, "Config Fault Time"=33693184, "Motor Ack"=33693696] ("CAN Motor Message IDs")
                n190 = call <vilib>:"WPI_CANJaguar_GetTransaction.vi"("error in"=w412, "Message ID"=w415, "CAN Jaguar Ref"=w418) -> ("error out"=w414:errorcluster, "Data Out"=w417:u8[], "CAN Jaguar Ref Out"=w413:T3)  [unwired: 6 out]
                n191 = Byte Array To String(unsigned byte array=w417) -> (string=w416:string)
                n192 = Unflatten From String(type=i16 0 ("Voltage"), binary string=w416, byte order (0:big-endian, network order)=w426, error in (no error)=w414) -> (value=w423:i16, error out=w424:errorcluster)  [unwired: 2 out]
                n193 = Divide(x=w423, y=256) -> (x/y=w419:dbl)
                n194 = Bundle By Name(cluster=w421, "Temperature"=w419) -> (w420:T2)
              }
              frame "Position" {
                w436 = T11 33690880 items=["Volt Enable"=33685504, "Volt Disable"=33685568, "Volt Set"=33685632, "Volt Set Ramp"=33685696, "Volt Set No Ack"=33686080, "Speed Enable"=33686528, "Speed Disable"=33686592, "Speed Set"=33686656, "Speed P"=33686720, "Speed I"=33686784, "Speed D"=33686848, "Speed Ref"=33686912, "Speed Set No Ack"=33687232, "Volt Comp Enable"=33687552, "Volt Comp Disable"=33687616, "Volt Comp Set"=33687680, "Volt Comp In Ramp"=33687744, "Volt Comp Comp Ramp"=33687808, "Volt Comp Set No Ack"=33688128, "Position Enable"=33688576, "Position Disable"=33688640, "Position Set"=33688704, "Position P"=33688768, "Position I"=33688832, "Position D"=33688896, "Position Ref"=33688960, "Position Set No Ack"=33689280, "Current Enable"=33689600, "Current Disable"=33689664, "Current Set"=33689728, "Current P"=33689792, "Current I"=33689856, "Current D"=33689920, "Current Set No Ack"=33690240, "Status Percent VBus"=33690624, "Status VBus"=33690688, "Status Current"=33690752, "Status Temp"=33690816, "Status Position"=33690880, "Status Speed"=33690944, "Status Limit"=33691008, "Status Fault"=33691072, "Status Power"=33691136, "Status Control Mode"=33691200, "Status VOut"=33691264, "Status Sticky Fault"=33691328, "Status Fault Count"=33691392, "Periodic Status Enable 0"=33691648, "Periodic Status Enable 1"=33691712, "Periodic Status Enable 2"=33691776, "Periodic Status Enable 3"=33691840, "Periodic Status Config 0"=33691904, "Periodic Status Config 1"=33691968, "Periodic Status Config 2"=33692032, "Periodic Status Config 3"=33692096, "Periodic Status Data 0"=33692160, "Periodic Status Data 1"=33692224, "Periodic Status Data 2"=33692288, "Periodic Status Data 3"=33692352, "Config Num Brushes"=33692672, "Config Encoder Lines"=33692736, "Config Pot Turns"=33692800, "Config Brake Coast"=33692864, "Config Limit Mode"=33692928, "Config Limit Fwd"=33692992, "Config Limit Rev"=33693056, "Config Max VOut"=33693120, "Config Fault Time"=33693184, "Motor Ack"=33693696] ("CAN Motor Message IDs")
                n195 = call <vilib>:"WPI_CANJaguar_GetTransaction.vi"("error in"=w432, "Message ID"=w436, "CAN Jaguar Ref"=w433) -> ("error out"=w435:errorcluster, "Data Out"=w434:u8[], "CAN Jaguar Ref Out"=w427:T3)  [unwired: 6 out]
                n196 = Byte Array To String(unsigned byte array=w434) -> (string=w437:string)
                n197 = Unflatten From String(type=0 ("Voltage"), binary string=w437, byte order (0:big-endian, network order)=w444, error in (no error)=w435) -> (value=w439:i32, error out=w442:errorcluster)  [unwired: 2 out]
                n198 = Unbundle By Name(w427) -> ("Invert"=w431:bool)
                n199 = Divide(x=w439, y=65536 ("value")) -> (x/y=w429:dbl)
                n200 = Negate(x=w429) -> (-x=w430:dbl)
                n201 = Select(t=w430, s=w431, f=w429) -> (s? t:f=w428:dbl)
                n202 = Bundle By Name(cluster=w441, "Position"=w428) -> (w440:T2)
              }
              frame "Speed" {
                w452 = T11 33690944 items=["Volt Enable"=33685504, "Volt Disable"=33685568, "Volt Set"=33685632, "Volt Set Ramp"=33685696, "Volt Set No Ack"=33686080, "Speed Enable"=33686528, "Speed Disable"=33686592, "Speed Set"=33686656, "Speed P"=33686720, "Speed I"=33686784, "Speed D"=33686848, "Speed Ref"=33686912, "Speed Set No Ack"=33687232, "Volt Comp Enable"=33687552, "Volt Comp Disable"=33687616, "Volt Comp Set"=33687680, "Volt Comp In Ramp"=33687744, "Volt Comp Comp Ramp"=33687808, "Volt Comp Set No Ack"=33688128, "Position Enable"=33688576, "Position Disable"=33688640, "Position Set"=33688704, "Position P"=33688768, "Position I"=33688832, "Position D"=33688896, "Position Ref"=33688960, "Position Set No Ack"=33689280, "Current Enable"=33689600, "Current Disable"=33689664, "Current Set"=33689728, "Current P"=33689792, "Current I"=33689856, "Current D"=33689920, "Current Set No Ack"=33690240, "Status Percent VBus"=33690624, "Status VBus"=33690688, "Status Current"=33690752, "Status Temp"=33690816, "Status Position"=33690880, "Status Speed"=33690944, "Status Limit"=33691008, "Status Fault"=33691072, "Status Power"=33691136, "Status Control Mode"=33691200, "Status VOut"=33691264, "Status Sticky Fault"=33691328, "Status Fault Count"=33691392, "Periodic Status Enable 0"=33691648, "Periodic Status Enable 1"=33691712, "Periodic Status Enable 2"=33691776, "Periodic Status Enable 3"=33691840, "Periodic Status Config 0"=33691904, "Periodic Status Config 1"=33691968, "Periodic Status Config 2"=33692032, "Periodic Status Config 3"=33692096, "Periodic Status Data 0"=33692160, "Periodic Status Data 1"=33692224, "Periodic Status Data 2"=33692288, "Periodic Status Data 3"=33692352, "Config Num Brushes"=33692672, "Config Encoder Lines"=33692736, "Config Pot Turns"=33692800, "Config Brake Coast"=33692864, "Config Limit Mode"=33692928, "Config Limit Fwd"=33692992, "Config Limit Rev"=33693056, "Config Max VOut"=33693120, "Config Fault Time"=33693184, "Motor Ack"=33693696] ("CAN Motor Message IDs")
                n203 = call <vilib>:"WPI_CANJaguar_GetTransaction.vi"("error in"=w450, "Message ID"=w452, "CAN Jaguar Ref"=w451) -> ("error out"=w453:errorcluster, "Data Out"=w454:u8[], "CAN Jaguar Ref Out"=w445:T3)  [unwired: 6 out]
                n204 = Byte Array To String(unsigned byte array=w454) -> (string=w455:string)
                n205 = Unflatten From String(type=0 ("Voltage"), binary string=w455, byte order (0:big-endian, network order)=w462, error in (no error)=w453) -> (value=w456:i32, error out=w460:errorcluster)  [unwired: 2 out]
                n206 = Unbundle By Name(w445) -> ("Invert"=w449:bool)
                n207 = Divide(x=w456, y=65536 ("value")) -> (x/y=w446:dbl)
                n208 = Negate(x=w446) -> (-x=w448:dbl)
                n209 = Select(t=w448, s=w449, f=w446) -> (s? t:f=w447:dbl)
                n210 = Bundle By Name(cluster=w459, "Speed"=w447) -> (w458:T2)
              }
              frame "Limit Switches" {
                w471 = T11 33691008 items=["Volt Enable"=33685504, "Volt Disable"=33685568, "Volt Set"=33685632, "Volt Set Ramp"=33685696, "Volt Set No Ack"=33686080, "Speed Enable"=33686528, "Speed Disable"=33686592, "Speed Set"=33686656, "Speed P"=33686720, "Speed I"=33686784, "Speed D"=33686848, "Speed Ref"=33686912, "Speed Set No Ack"=33687232, "Volt Comp Enable"=33687552, "Volt Comp Disable"=33687616, "Volt Comp Set"=33687680, "Volt Comp In Ramp"=33687744, "Volt Comp Comp Ramp"=33687808, "Volt Comp Set No Ack"=33688128, "Position Enable"=33688576, "Position Disable"=33688640, "Position Set"=33688704, "Position P"=33688768, "Position I"=33688832, "Position D"=33688896, "Position Ref"=33688960, "Position Set No Ack"=33689280, "Current Enable"=33689600, "Current Disable"=33689664, "Current Set"=33689728, "Current P"=33689792, "Current I"=33689856, "Current D"=33689920, "Current Set No Ack"=33690240, "Status Percent VBus"=33690624, "Status VBus"=33690688, "Status Current"=33690752, "Status Temp"=33690816, "Status Position"=33690880, "Status Speed"=33690944, "Status Limit"=33691008, "Status Fault"=33691072, "Status Power"=33691136, "Status Control Mode"=33691200, "Status VOut"=33691264, "Status Sticky Fault"=33691328, "Status Fault Count"=33691392, "Periodic Status Enable 0"=33691648, "Periodic Status Enable 1"=33691712, "Periodic Status Enable 2"=33691776, "Periodic Status Enable 3"=33691840, "Periodic Status Config 0"=33691904, "Periodic Status Config 1"=33691968, "Periodic Status Config 2"=33692032, "Periodic Status Config 3"=33692096, "Periodic Status Data 0"=33692160, "Periodic Status Data 1"=33692224, "Periodic Status Data 2"=33692288, "Periodic Status Data 3"=33692352, "Config Num Brushes"=33692672, "Config Encoder Lines"=33692736, "Config Pot Turns"=33692800, "Config Brake Coast"=33692864, "Config Limit Mode"=33692928, "Config Limit Fwd"=33692992, "Config Limit Rev"=33693056, "Config Max VOut"=33693120, "Config Fault Time"=33693184, "Motor Ack"=33693696] ("CAN Motor Message IDs")
                n211 = call <vilib>:"WPI_CANJaguar_GetTransaction.vi"("error in"=w469, "Message ID"=w471, "CAN Jaguar Ref"=w472) -> ("error out"=w474:errorcluster, "Data Out"=w473:u8[], "CAN Jaguar Ref Out"=w470:T3)  [unwired: 6 out]
                n212 = Byte Array To String(unsigned byte array=w473) -> (string=w475:string)
                n213 = Unflatten From String(type=u8 0 ("Voltage"), binary string=w475, byte order (0:big-endian, network order)=w484, error in (no error)=w474) -> (value=w479:u8, error out=w482:errorcluster)  [unwired: 2 out]
                n214 = Number To Boolean Array(number=w479) -> (Boolean array=w478:bool[])
                n215 = Index Array(array=w478) -> (element #1=w477:bool, element #2=w476:bool, element #3=w468:bool, element #4=w467:bool, element #5=w466:bool, element #6=w465:bool, element #7=w464:bool, element #8=w463:bool)  [unwired: 8 in]
                n216 = Bundle By Name(cluster=w481, "Limits.Forward Limit"=w477, "Limits.Reverse Limit"=w476, "Limits.Forward Soft Limit"=w468, "Limits.Reverse Soft Limit"=w467, "Limits.Sticky Forward Limit"=w466, "Limits.Sticky Reverse Limit"=w465, "Limits.Sticky Forward Soft Limit"=w464, "Limits.Sticky Reverse Soft Limit"=w463) -> (w480:T2)
              }
              frame "Faults" {
                w487 = T11 33691328 items=["Volt Enable"=33685504, "Volt Disable"=33685568, "Volt Set"=33685632, "Volt Set Ramp"=33685696, "Volt Set No Ack"=33686080, "Speed Enable"=33686528, "Speed Disable"=33686592, "Speed Set"=33686656, "Speed P"=33686720, "Speed I"=33686784, "Speed D"=33686848, "Speed Ref"=33686912, "Speed Set No Ack"=33687232, "Volt Comp Enable"=33687552, "Volt Comp Disable"=33687616, "Volt Comp Set"=33687680, "Volt Comp In Ramp"=33687744, "Volt Comp Comp Ramp"=33687808, "Volt Comp Set No Ack"=33688128, "Position Enable"=33688576, "Position Disable"=33688640, "Position Set"=33688704, "Position P"=33688768, "Position I"=33688832, "Position D"=33688896, "Position Ref"=33688960, "Position Set No Ack"=33689280, "Current Enable"=33689600, "Current Disable"=33689664, "Current Set"=33689728, "Current P"=33689792, "Current I"=33689856, "Current D"=33689920, "Current Set No Ack"=33690240, "Status Percent VBus"=33690624, "Status VBus"=33690688, "Status Current"=33690752, "Status Temp"=33690816, "Status Position"=33690880, "Status Speed"=33690944, "Status Limit"=33691008, "Status Fault"=33691072, "Status Power"=33691136, "Status Control Mode"=33691200, "Status VOut"=33691264, "Status Sticky Fault"=33691328, "Status Fault Count"=33691392, "Periodic Status Enable 0"=33691648, "Periodic Status Enable 1"=33691712, "Periodic Status Enable 2"=33691776, "Periodic Status Enable 3"=33691840, "Periodic Status Config 0"=33691904, "Periodic Status Config 1"=33691968, "Periodic Status Config 2"=33692032, "Periodic Status Config 3"=33692096, "Periodic Status Data 0"=33692160, "Periodic Status Data 1"=33692224, "Periodic Status Data 2"=33692288, "Periodic Status Data 3"=33692352, "Config Num Brushes"=33692672, "Config Encoder Lines"=33692736, "Config Pot Turns"=33692800, "Config Brake Coast"=33692864, "Config Limit Mode"=33692928, "Config Limit Fwd"=33692992, "Config Limit Rev"=33693056, "Config Max VOut"=33693120, "Config Fault Time"=33693184, "Motor Ack"=33693696] ("CAN Motor Message IDs")
                n217 = call <vilib>:"WPI_CANJaguar_GetTransaction.vi"("error in"=w491, "Message ID"=w487, "CAN Jaguar Ref"=w492) -> ("error out"=w494:errorcluster, "Data Out"=w493:u8[], "CAN Jaguar Ref Out"=w486:T3)  [unwired: 6 out]
                n218 = Byte Array To String(unsigned byte array=w493) -> (string=w495:string)
                n219 = Unflatten From String(type=u16 0 ("Voltage"), binary string=w495, byte order (0:big-endian, network order)=w503, error in (no error)=w494) -> (value=w499:u16, error out=w485:errorcluster)  [unwired: 2 out]
                n220 = Number To Boolean Array(number=w499) -> (Boolean array=w488:bool[])
                n221 = Index Array(array=w488) -> (element #1=w498:bool, element #2=w497:bool, element #3=w496:bool, element #4=w490:bool, element #5=w489:bool)  [unwired: 5 in]
                n222 = Bundle By Name(cluster=w501, "Faults.Current Fault"=w498, "Faults.Temperature Fault"=w497, "Faults.Bus Voltage Fault"=w496, "Faults.Gate Driver Fault"=w490, "Faults.Comm Fault"=w489) -> (w500:T2)
              }
              frame "Fault Counters" {
                w505 = T11 33691392 items=["Volt Enable"=33685504, "Volt Disable"=33685568, "Volt Set"=33685632, "Volt Set Ramp"=33685696, "Volt Set No Ack"=33686080, "Speed Enable"=33686528, "Speed Disable"=33686592, "Speed Set"=33686656, "Speed P"=33686720, "Speed I"=33686784, "Speed D"=33686848, "Speed Ref"=33686912, "Speed Set No Ack"=33687232, "Volt Comp Enable"=33687552, "Volt Comp Disable"=33687616, "Volt Comp Set"=33687680, "Volt Comp In Ramp"=33687744, "Volt Comp Comp Ramp"=33687808, "Volt Comp Set No Ack"=33688128, "Position Enable"=33688576, "Position Disable"=33688640, "Position Set"=33688704, "Position P"=33688768, "Position I"=33688832, "Position D"=33688896, "Position Ref"=33688960, "Position Set No Ack"=33689280, "Current Enable"=33689600, "Current Disable"=33689664, "Current Set"=33689728, "Current P"=33689792, "Current I"=33689856, "Current D"=33689920, "Current Set No Ack"=33690240, "Status Percent VBus"=33690624, "Status VBus"=33690688, "Status Current"=33690752, "Status Temp"=33690816, "Status Position"=33690880, "Status Speed"=33690944, "Status Limit"=33691008, "Status Fault"=33691072, "Status Power"=33691136, "Status Control Mode"=33691200, "Status VOut"=33691264, "Status Sticky Fault"=33691328, "Status Fault Count"=33691392, "Periodic Status Enable 0"=33691648, "Periodic Status Enable 1"=33691712, "Periodic Status Enable 2"=33691776, "Periodic Status Enable 3"=33691840, "Periodic Status Config 0"=33691904, "Periodic Status Config 1"=33691968, "Periodic Status Config 2"=33692032, "Periodic Status Config 3"=33692096, "Periodic Status Data 0"=33692160, "Periodic Status Data 1"=33692224, "Periodic Status Data 2"=33692288, "Periodic Status Data 3"=33692352, "Config Num Brushes"=33692672, "Config Encoder Lines"=33692736, "Config Pot Turns"=33692800, "Config Brake Coast"=33692864, "Config Limit Mode"=33692928, "Config Limit Fwd"=33692992, "Config Limit Rev"=33693056, "Config Max VOut"=33693120, "Config Fault Time"=33693184, "Motor Ack"=33693696] ("CAN Motor Message IDs")
                # "Reset all fault counters"
                n223 = call <vilib>:"WPI_CANJaguar_GetTransaction.vi"("error in"=w516, "Message ID"=w505, "CAN Jaguar Ref"=w517) -> ("error out"=w508:errorcluster, "Data Out"=w513:u8[], "CAN Jaguar Ref Out"=w506:T3)  [unwired: 6 out]
                n224 = Index Array(array=w513) -> (element #1=w520:u8, element #2=w519:u8, element #3=w518:u8, element #4=w515:u8, element #5=w514:u8, element #6=w511:u8, element #7=w510:u8, element #8=w512:u8)  [unwired: 8 in]
                n225 = Bundle By Name(cluster=w522, "Fault Counters.Current Faults"=w520, "Fault Counters.Temperature Faults"=w519, "Fault Counters.Bus Voltage Faults"=w518, "Fault Counters.Gate Driver Faults"=w515, "Fault Counters.Comm Faults"=w514, "Fault Counters.CAN Status"=w511, "Fault Counters.CAN RX Errors"=w510, "Fault Counters.CAN TX Errors"=w512) -> (w521:T2)
                n226 = call <vilib>:"WPI_CANJaguar_SetTransaction.vi"("error in"=w508, "Data"=u8[] [63] ("data"), "Message ID"=w505, "CAN Jaguar Ref"=w506) -> ("error out"=w507:errorcluster, "CAN Jaguar Ref Out"=w504:T3)  [unwired: 6 out]
              }
              frame "Power Cycle" {
                w536 = T11 33691136 items=["Volt Enable"=33685504, "Volt Disable"=33685568, "Volt Set"=33685632, "Volt Set Ramp"=33685696, "Volt Set No Ack"=33686080, "Speed Enable"=33686528, "Speed Disable"=33686592, "Speed Set"=33686656, "Speed P"=33686720, "Speed I"=33686784, "Speed D"=33686848, "Speed Ref"=33686912, "Speed Set No Ack"=33687232, "Volt Comp Enable"=33687552, "Volt Comp Disable"=33687616, "Volt Comp Set"=33687680, "Volt Comp In Ramp"=33687744, "Volt Comp Comp Ramp"=33687808, "Volt Comp Set No Ack"=33688128, "Position Enable"=33688576, "Position Disable"=33688640, "Position Set"=33688704, "Position P"=33688768, "Position I"=33688832, "Position D"=33688896, "Position Ref"=33688960, "Position Set No Ack"=33689280, "Current Enable"=33689600, "Current Disable"=33689664, "Current Set"=33689728, "Current P"=33689792, "Current I"=33689856, "Current D"=33689920, "Current Set No Ack"=33690240, "Status Percent VBus"=33690624, "Status VBus"=33690688, "Status Current"=33690752, "Status Temp"=33690816, "Status Position"=33690880, "Status Speed"=33690944, "Status Limit"=33691008, "Status Fault"=33691072, "Status Power"=33691136, "Status Control Mode"=33691200, "Status VOut"=33691264, "Status Sticky Fault"=33691328, "Status Fault Count"=33691392, "Periodic Status Enable 0"=33691648, "Periodic Status Enable 1"=33691712, "Periodic Status Enable 2"=33691776, "Periodic Status Enable 3"=33691840, "Periodic Status Config 0"=33691904, "Periodic Status Config 1"=33691968, "Periodic Status Config 2"=33692032, "Periodic Status Config 3"=33692096, "Periodic Status Data 0"=33692160, "Periodic Status Data 1"=33692224, "Periodic Status Data 2"=33692288, "Periodic Status Data 3"=33692352, "Config Num Brushes"=33692672, "Config Encoder Lines"=33692736, "Config Pot Turns"=33692800, "Config Brake Coast"=33692864, "Config Limit Mode"=33692928, "Config Limit Fwd"=33692992, "Config Limit Rev"=33693056, "Config Max VOut"=33693120, "Config Fault Time"=33693184, "Motor Ack"=33693696] ("CAN Motor Message IDs")
                n227 = call <vilib>:"WPI_CANJaguar_GetTransaction.vi"("error in"=w527, "Message ID"=w536, "CAN Jaguar Ref"=w531) -> ("error out"=w526:errorcluster, "Data Out"=w537:u8[], "CAN Jaguar Ref Out"=w529:T3)  [unwired: 6 out]
                n228 = Byte Array To String(unsigned byte array=w537) -> (string=w533:string)
                n229 = Unflatten From String(type=u8 0 ("Voltage"), binary string=w533, byte order (0:big-endian, network order)=w530, error in (no error)=w526) -> (value=w532:u8, error out=w525:errorcluster)  [unwired: 2 out]
                n230 = Not Equal To 0?(x=w532) -> (x != 0?=w523:bool)
                n231 = Bundle By Name(cluster=w539, "Power Cycle"=w523) -> (w538:T2)
                n232 = case shown="True" w523 {
                  tunnel: w536 -> [_ w547]
                  tunnel: u8[] [1] ("data") -> [_ w546]
                  tunnel: w529 -> [w541 w545]
                  tunnel: [w541 w544] -> w528
                  tunnel: w525 -> [w540 w543]
                  tunnel: [w540 w542] -> w524
                  frame False {
                  }
                  frame True {
                    n233 = call <vilib>:"WPI_CANJaguar_SetTransaction.vi"("error in"=w543, "Data"=w546, "Message ID"=w547, "CAN Jaguar Ref"=w545) -> ("error out"=w542:errorcluster, "CAN Jaguar Ref Out"=w544:T3)  [unwired: 6 out]
                  }
                }
              }
            }
          }
        }
      }
    }
    frame Error {
    }
  }
  "CAN Jaguar Ref" <- w8
  "error out" <- w6
  "Status" <- w3
